vi "Destroy Events.vi"(8 "error in (no error)":errorcluster, 11 "DAQ_Engine in":refnum<class "DAQ_Engine.lvclass">) -> (0 "error out":errorcluster, 3 "DAQ_Engine out":refnum<class "DAQ_Engine.lvclass">)   [LabVIEW 2019, in "DAQ_Engine.lvclass"]
doc: "Developed by Kevin Thompson\nkevin@thompsonengineering.net\n\nCopyright 2018\nThompson Engineering, LLC"
uses:
  DAQ_Engine.lvclass
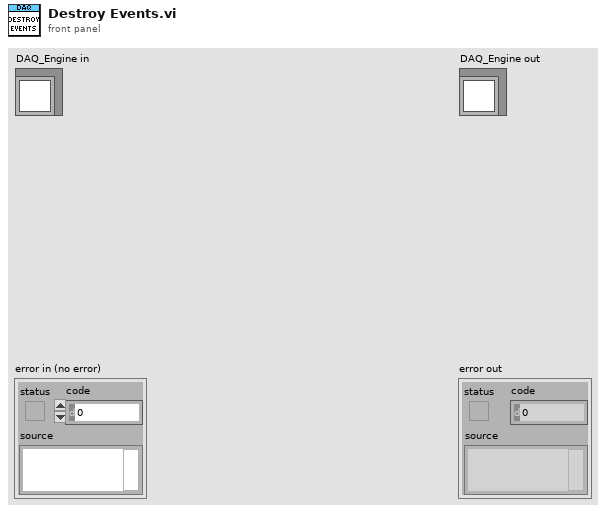
[diagram p1: front panel]
types:
  T1 = typedef "DAQ_Engine.lvclass/Public Events--cluster.ctl" = cluster{"DAQ_Engine.AsyncCmd Event":refnum<user-event>, "DAQ_Engine.AsyncMsg Event":refnum<user-event>, "stop process":refnum<user-event>, "DAQ_Engine.DAQStateChg Ev":refnum<user-event>, "DAQ_Engine.MeasSettingsChg Ev":refnum<user-event>, "DAQ_Engine.AcqModeChg Ev":refnum<user-event>}
  T2 = typedef "DAQ_Engine.lvclass/ObjData--cluster.ctl" = cluster{"Settings":T3, "Public Events":T1, "Dependency":T8, "ReadData-placeholder":T9, "VISA-placeholder":refnum<visa-resource-name>, "MeasSettings":T4, "InverterDataAcqMode":T7, "RawDaqDataQ":T10, "Private Events":T11, "DAQState Data":T12}
  T3 = typedef "DAQ_Engine.lvclass/Settings--cluster.ctl" = cluster{"Simulation":bool, "Initial ErrReporting setting":i32, "Initial Measurement settings":T4, "BoardNum":T6, "Acquisition mode":T7, "DemoMode":bool}
  T4 = typedef "Measurement Config--cluster.ctl" = cluster{"Data Rate 9775":T5, "Data Rate 9215":u32, "Samples RMS 9215":u32, "Samples RMS 9775":u32}
  T5 = typedef "nicrio_cRIO-9775_ContinuousDataRates4ChansRing.ctl" = u16
  T6 = typedef "DAQ_Engine.lvclass/BoardNum--cluster.ctl" = cluster{"P1Sgl":u32, "P2":u32, "P3":u32}
  T7 = typedef "Acquisition Mode--cluster.ctl" = enum16{"3phase", "Single"}
  T8 = typedef "DAQ_Engine.lvclass/Dependency--cluster.ctl" = cluster{"Config":refnum<class "Config.lvclass">}
  T9 = typedef "DAQ_Engine.lvclass/Read Data--cluster.ctl" = cluster{"Data":dbl}
  T10 = typedef "RawDAQDataQRef--cluster.ctl" = refnum<queue>
  T11 = typedef "DAQ_Engine.lvclass/Private Events--cluster.ctl" = cluster{"PrivateAsync Ev":refnum<user-event>}
  T12 = typedef "DAQ_Engine.lvclass/DAQStateEvData--cluster.ctl" = cluster{"DAQState":T13, "vData":variant}
  T13 = typedef "DAQState--enum.ctl" = enum16{"Unknown", "Stopped", "Running", "Error"}
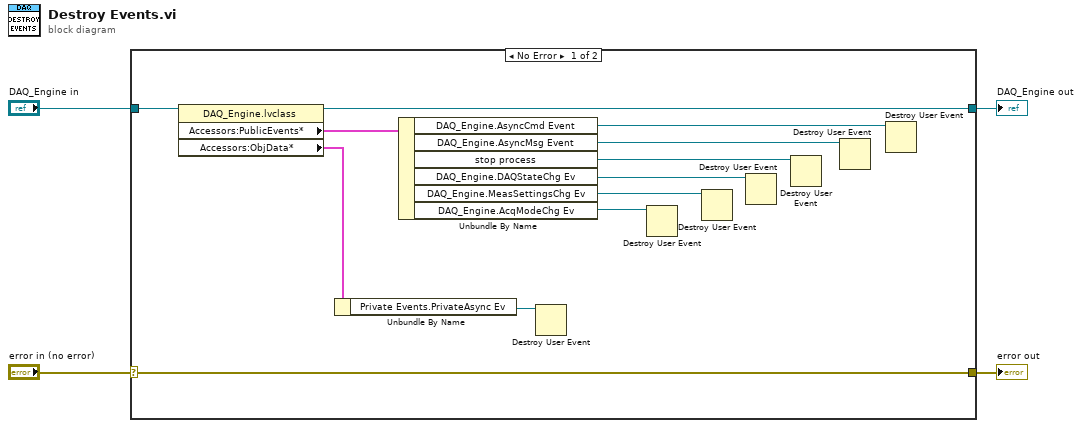
[diagram p0: block diagram]
diagram:
  n1 = case shown="No Error" "error in (no error)" {
    selector: "error in (no error)" -> [w12 w18]
    tunnel: [w12 w18] -> w3
    tunnel: [w15 w17] -> w1
    tunnel: "DAQ_Engine in" -> [w16 w17]
    frame No Error {
      n2 = property class="DAQ_Engine.lvclass"(reference=w16) -> (reference out=w15:refnum<class "DAQ_Engine.lvclass">, "Accessors:PublicEvents*"=w14:T1, "Accessors:ObjData*"=w7:T2)  [unwired: 1 in, 1 out]
      n3 = Unbundle By Name(w7) -> ("Private Events.PrivateAsync Ev"=w8:refnum<user-event>)
      n4 = Unbundle By Name(w14) -> ("DAQ_Engine.AsyncCmd Event"=w13:refnum<user-event>, "DAQ_Engine.AsyncMsg Event"=w11:refnum<user-event>, "stop process"=w10:refnum<user-event>, "DAQ_Engine.DAQStateChg Ev"=w9:refnum<user-event>, "DAQ_Engine.MeasSettingsChg Ev"=w5:refnum<user-event>, "DAQ_Engine.AcqModeChg Ev"=w6:refnum<user-event>)
      n5 = Destroy User Event(user event=w8) -> ()  [unwired: 1 in, 1 out]
      n6 = Destroy User Event(user event=w6) -> ()  [unwired: 1 in, 1 out]
      n7 = Destroy User Event(user event=w5) -> ()  [unwired: 1 in, 1 out]
      n8 = Destroy User Event(user event=w9) -> ()  [unwired: 1 in, 1 out]
      n9 = Destroy User Event(user event=w10) -> ()  [unwired: 1 in, 1 out]
      n10 = Destroy User Event(user event=w11) -> ()  [unwired: 1 in, 1 out]
      n11 = Destroy User Event(user event=w13) -> ()  [unwired: 1 in, 1 out]
    }
    frame Error {
    }
  }
  "error out" <- w3
  "DAQ_Engine out" <- w1
